vi "SetFileMethod.vi"(0 "object in":refnum<class "Client.lvclass">, 1 "File Method":T1, 5 "Error In":errorcluster) -> (14 "object out":refnum<class "Client.lvclass">, 19 "Error Out":errorcluster)   [LabVIEW 2024, in "Client.lvclass"]
uses:
  Client.lvclass
  Support/Type Def/File Method.ctl
  Implementations/Logger/Logger.lvclass
  C:/Users/burakkorkmaz/Desktop/Leveling/labview-desing-patterns/Bridge Pattern/IDataMethod_interface/IDataMethod.lvclass
  Implementations/Viewer/Viewer.lvclass
  Client.lvclass/Client.ctl
  Abstractions/DataType/DataType.lvclass
panel:
  # "Connector Pane"
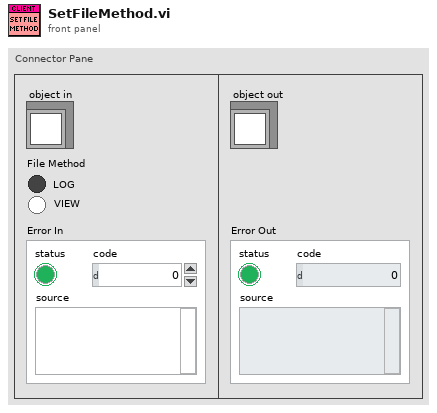
[diagram p1: front panel]
types:
  T1 = typedef "File Method.ctl" = enum32{"Log", "View"}
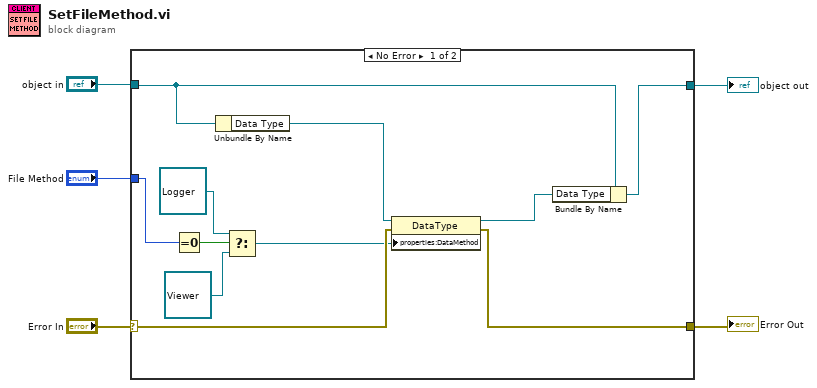
[diagram p0: block diagram]
diagram:
  n1 = case shown="No Error" "Error In" {
    selector: "Error In" -> [w13 w18]
    tunnel: [w12 w18] -> w4
    tunnel: [w16 w17] -> w2
    tunnel: "object in" -> [w15 w17]
    tunnel: "File Method" -> [w9 _]
    frame No Error {
      n2 = Equal To 0?(x=w9) -> (x = 0?=w10:bool)
      n3 = Unbundle By Name(w15) -> ("Data Type"=w14:refnum<class "DataType.lvclass">)
      n4 = Select(t=refnum<class "Logger.lvclass"> refnum ("Logger"), s=w10, f=refnum<class "Viewer.lvclass"> refnum ("Viewer")) -> (s? t:f=w6:refnum<class "IDataMethod.lvclass">)
      n5 = property class="DataType"(reference=w14, error in=w13, "properties:DataMethod"=w6) -> (reference out=w11:refnum<class "DataType.lvclass">, error out=w12:errorcluster)
      n6 = Bundle By Name(cluster=w15, "Data Type"=w11) -> (w16:refnum<class "Client.lvclass">)
    }
    frame Error {
    }
  }
  "Error Out" <- w4
  "object out" <- w2
